vi "Horizontal MenuList_Init.vi"(3 "Container State":T4, 4 "Previous State":variant, 5 "Previous Version":T3) -> (2 "Current State":T1={"Persistent"={"Elements"=[], "PicElements"=[], "Limits"=[], "Selection"=[], "Selection Color"=4359423, "Highlight"=[], "Highlight Val"=-1, "Highlight Color"={"Back"=12966892, "Edge"=4359423}, "Font"={"Details"={"Font Name:"="Segoe UI", "Size"=18, "Strikeout?"=FALSE, "Italic?"=FALSE, "Underline?"=FALSE, "Outline?"=FALSE, "Shadow?"=FALSE, "Bold?"=TRUE}, "Color"=3289650}, "Bakground Color"=0}, "List Ref"=refnum, "nbVisible"=0, "FirstIdx"=0, "More.Width"=0})   [LabVIEW 2016, in "Horizontal MenuList.xctl"]
uses:
  Horizontal MenuList.xctl
  Horizontal MenuList_State.ctl
  _SubVIs/Highlight Colors.ctl
  <vilib>/_xctls/Container State.ctl
  <vilib>/_xctls/Version.ctl
  <vilib>/_xctls/XControlSupport.lvlib
panel:
  in  "Default":T1={"Persistent"={"Elements"=["Welcome", "System", "Dashboard", "Settings", "Help"], "PicElements"=[bytes[74], bytes[72], bytes[76], bytes[74], bytes[70]], "Limits"=[0, 90, 164, 267, 349, 403], "Selection"=[bytes[38], bytes[38], bytes[38], bytes[38], bytes[38]], "Selection Color"=2782463, "Highlight"=[bytes[76], bytes[76], bytes[76], bytes[76], bytes[76]], "Highlight Val"=-1, "Highlight Color"={"Back"=12966380, "Edge"=2782463}, "Font"={"Details"={"Font Name:"="Segoe UI", "Size"=24, "Strikeout?"=FALSE, "Italic?"=FALSE, "Underline?"=FALSE, "Outline?"=FALSE, "Shadow?"=FALSE, "Bold?"=TRUE}, "Color"=6579300}, "Bakground Color"=0}, "List Ref"=refnum, "nbVisible"=0, "FirstIdx"=0, "More.Width"=0}
  in  "Default Indicator State":T1={"Persistent"={"Elements"=[], "PicElements"=[], "Limits"=[], "Selection"=[], "Selection Color"=0, "Highlight"=[], "Highlight Val"=0, "Highlight Color"={"Back"=0, "Edge"=0}, "Font"={"Details"={"Font Name:"="Lucida Sans", "Size"=24, "Strikeout?"=FALSE, "Italic?"=FALSE, "Underline?"=FALSE, "Outline?"=FALSE, "Shadow?"=FALSE, "Bold?"=TRUE}, "Color"=7697781}, "Bakground Color"=0}, "List Ref"=refnum, "nbVisible"=0, "FirstIdx"=0, "More.Width"=0}
  in  "Default Control State":T1={"Persistent"={"Elements"=[], "PicElements"=[], "Limits"=[], "Selection"=[], "Selection Color"=4359423, "Highlight"=[], "Highlight Val"=-1, "Highlight Color"={"Back"=12966892, "Edge"=4359423}, "Font"={"Details"={"Font Name:"="Segoe UI", "Size"=24, "Strikeout?"=FALSE, "Italic?"=FALSE, "Underline?"=FALSE, "Outline?"=FALSE, "Shadow?"=FALSE, "Bold?"=TRUE}, "Color"=3289650}, "Bakground Color"=0}, "List Ref"=refnum, "nbVisible"=0, "FirstIdx"=0, "More.Width"=0}
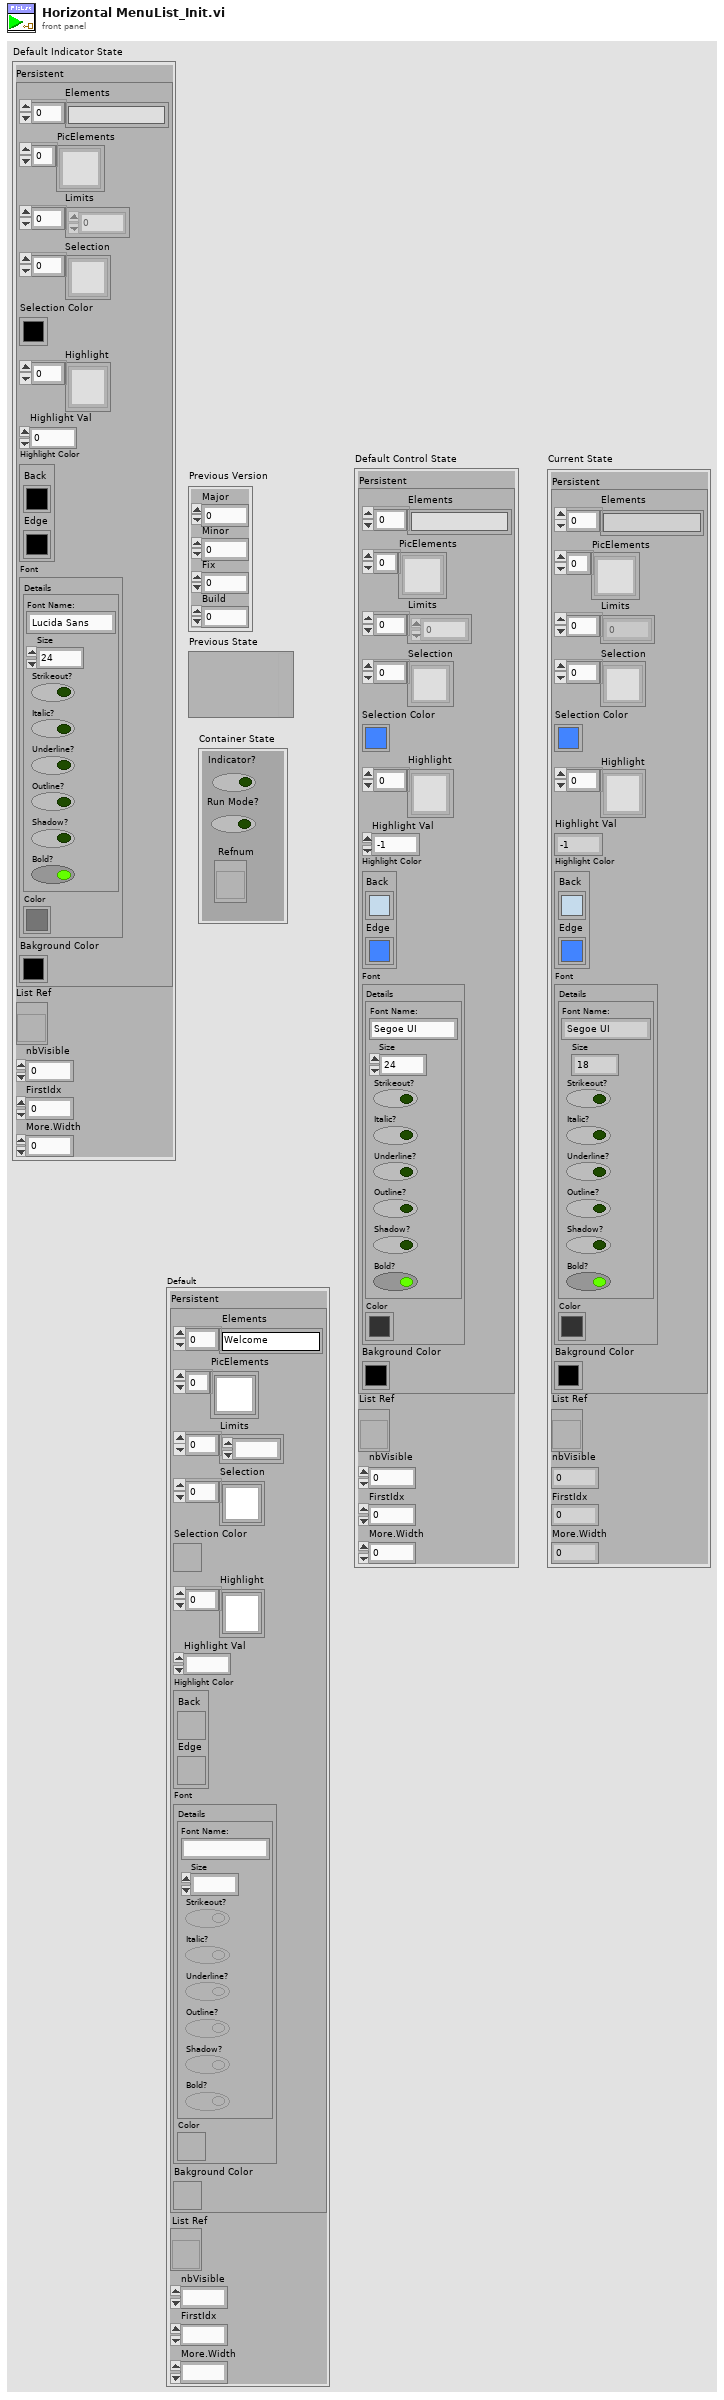
[diagram p1: front panel]
types:
  T1 = typedef "Horizontal MenuList.xctl/Horizontal MenuList_State.ctl" = cluster{"Persistent":cluster{"Elements":string[], "PicElements":picture[], "Limits":i32[], "Selection":picture[], "Selection Color":u32, "Highlight":picture[], "Highlight Val":i32, "Highlight Color":T2, "Font":cluster{"Details":cluster{"Font Name:":string, "Size":i16, "Strikeout?":bool, "Italic?":bool, "Underline?":bool, "Outline?":bool, "Shadow?":bool, "Bold?":bool}, "Color":u32}, "Bakground Color":u32}, "List Ref":refnum<vi>, "nbVisible":u8, "FirstIdx":u8, "More.Width":u8}
  T2 = typedef "Horizontal MenuList.xctl/Highlight Colors.ctl" = cluster{"Back":u32, "Edge":u32}
  T3 = typedef "XControlSupport.lvlib/Version.ctl" = cluster{"Major":u16, "Minor":u16, "Fix":u16, "Build":u16}
  T4 = typedef "XControlSupport.lvlib/Container State.ctl" = cluster{"Indicator?":bool, "Run Mode?":bool, " Refnum":refnum<vi>}
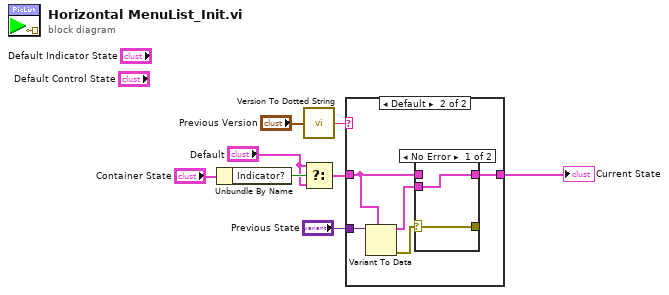
[diagram p0: block diagram]
diagram:
  n1 = Unbundle By Name("Container State") -> ("Indicator?"=w6:bool)
  n2 = call <vilib>:"Version To Dotted String.vi"("Version"="Previous Version") -> ("String Version"=w3:string)
  n3 = Select(t="Default", s=w6, f="Default") -> (s? t:f=w5:T1)
  n4 = case shown="Default" w3 {
    tunnel: "Previous State" -> [_ w14]
    tunnel: [w9 w10] -> w2
    tunnel: w5 -> [w9 w11]
    frame "0.0.0.0" {
    }
    frame Default {
      n5 = Variant To Data(type=w11, Variant=w14) -> (data=w12:T1, error out=w13:errorcluster)  [unwired: 1 in]
      n6 = case shown="No Error" w13 {
        selector: w13 -> [w16 w17]
        tunnel: w12 -> [w15 _]
        tunnel: [w15 w18] -> w10
        tunnel: w11 -> [_ w18]
        tunnel: [w16 w17] -> _
        frame No Error {
        }
        frame Error {
        }
      }
    }
  }
  "Current State" <- w2
